vi "Record Single Channel.vi"() -> ()   [LabVIEW 2014]
uses:
  <vilib>/DAQmx/read.llb/DAQmx Read (Analog 1D DBL 1Chan NSamp).vi
  <vilib>/DAQmx/create/channels.llb/DAQmx Create Channel (AI-Voltage-Basic).vi
  <vilib>/DAQmx/configure/timing.llb/DAQmx Timing (Sample Clock).vi
panel:
  in  "Record time per file (s)":dbl
  out "x >= y?":bool
  in  "File name add to the end \n(height)":string="h300"
  out "Sampling rate after filtering (Hz)":dbl
  in  "Avg points":i32
  in  "Filter type":T1(ring)
  in  "avg time (s)":dbl
  out "x/y":dbl
  in  "stop":bool
  in  "Record time (s)":dbl=1000.0 format="%0.2f"
  in  "Tab Control":enum32{"Page 1", "Page 2", "PSD", "PSD 2"}(tab)
  out "Waveform Chart":dbl[](graph)
  out "Waveform Graph":dbl[](graph)
  out "XY Graph":T2(graph)
  out "Waveform Graph 2":dbl[][](graph)
  in  "Save?":bool
  in  "number of samples per channel":i32=200000
  in  "rate":dbl=200000.0 format="%0.2f"
  in  "Sampling range (V)":dbl=1.0 format="%0.2f"
  in  "physical channels":tag="Dev2/ai19"
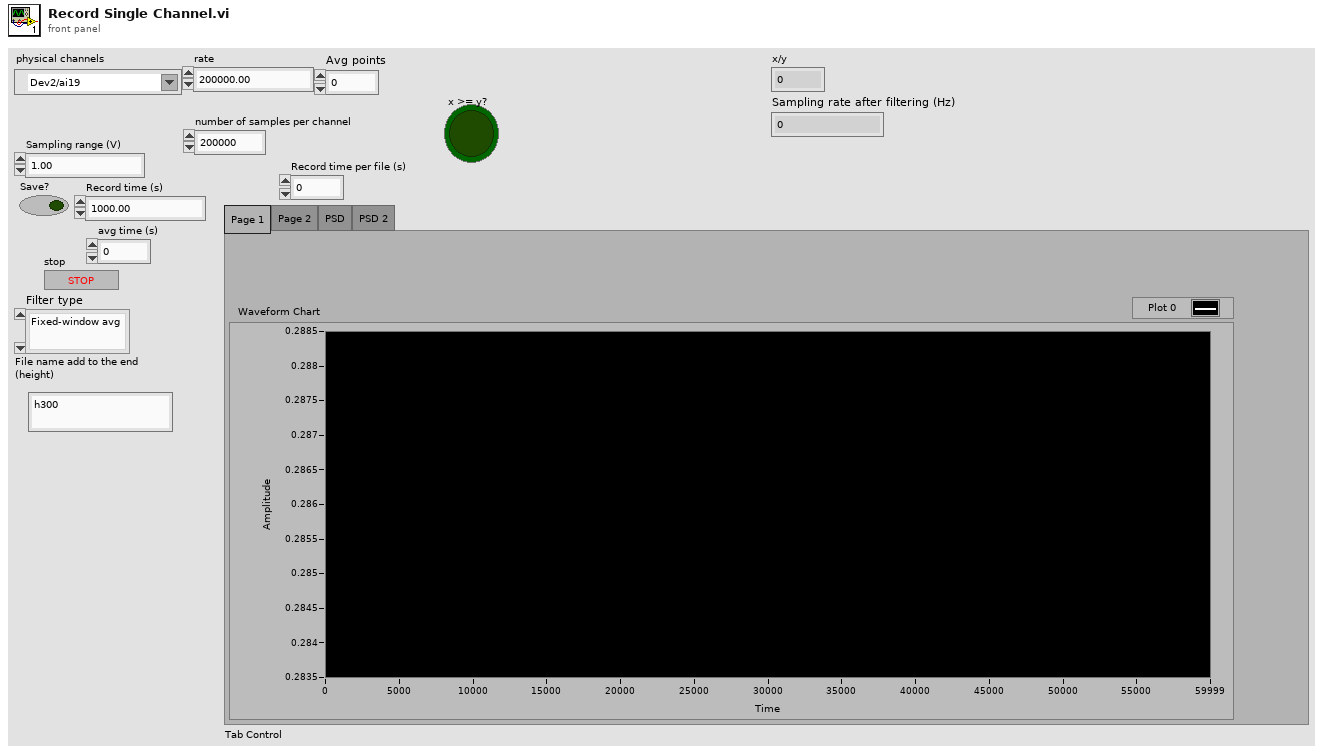
[diagram p1: front panel]
types:
  T1 = enum16{"Fixed-window avg", "Moving-window avg", "S-G filter", "Fixed-window Median", "Moving-window Median "}
  T2 = cluster{"Frequency (Hz)\n0,df, 2df,...(n/2-1)Fs":dbl[], "Avg. PSD":dbl[]}
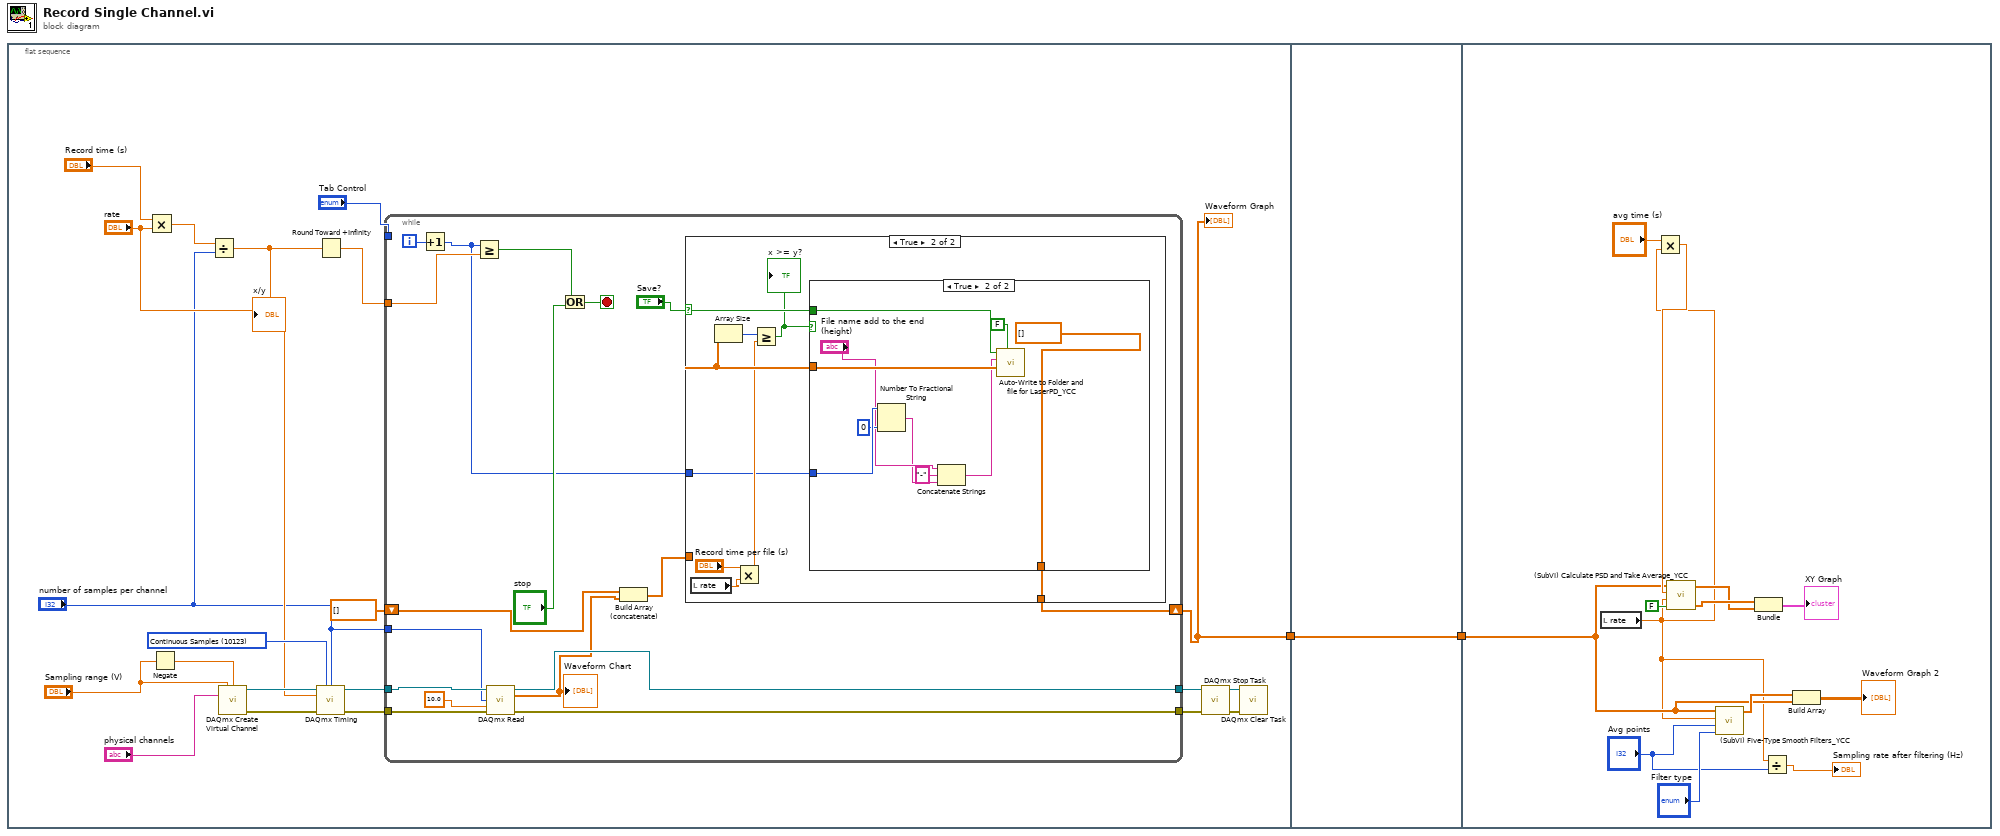
[diagram p0: block diagram]
diagram:
  n1 = flat-sequence {
    tunnel: [w3] -> w2
    tunnel: w2 -> [w62]
    tunnel: [w62] -> w1
    tunnel: w1 -> [w67]
    frame #0 {
      w18 = 10123 items=["Finite Samples"=10178, "Continuous Samples"=10123, "Hardware Timed Single Point"=12522] ("sample mode")
      n2 = Multiply(x="Record time (s)", y="rate") -> (x*y=w8:dbl)
      n3 = Negate(x="Sampling range (V)") -> (-x=w19:dbl)
      n4 = Divide(x=w8, y="number of samples per channel") -> (x/y=w7:dbl)
      "x/y" <- w7
      n5 = call-poly <vilib>:"DAQmx Create Virtual Channel.vi"("maximum value"="Sampling range (V)", "minimum value"=w19, "physical channels"="physical channels") -> ("task out"=w21:refnum<k21>, "error out"=w22:errorcluster)  [unwired: 11 in]
      n6 = Round Toward +Infinity(x=w7) -> (ceil(x): smallest int >= x=w6:dbl)
      n7 = call-poly <vilib>:"DAQmx Timing.vi"("task/channels in"=w21, "sample mode"=w18, "samples per channel"="number of samples per channel", "rate"="rate", "error in"=w22) -> ("task out"=w17:refnum<k21>, "error out"=w16:errorcluster)  [unwired: 9 in]
      n8 = while {
        tunnel: w17 -> [w40]
        tunnel: w16 -> [w39]
        tunnel: [w37] -> w15
        tunnel: [w36] -> w13
        tunnel: "Tab Control" -> [_]
        tunnel: w6 -> [w34]
        tunnel: "number of samples per channel" -> [w30]
        shift-right: [w25] -> w3
        shift-left: dbl[] [] -> [w28]
        i -> [w35]
        stop <- w31 stop-if-true
        n9 = Increment(x=w35) -> (x+1=w24:i32)
        n10 = Greater Or Equal?(x=w24, y=w34) -> (x >= y?=w33:bool)
        n11 = call-poly <vilib>:"DAQmx Read.vi"("task/channels in"=w40, "number of samples per channel"=w30, "timeout"=10.0, "error in"=w39) -> ("task out"=w37:refnum<k21>, "data"=w29:dbl[], "error out"=w36:errorcluster)  [unwired: 9 in]
        "Waveform Chart" <- w29
        n12 = Or(x=w33, y="stop") -> (x .or. y?=w31:bool)
        n13 = Build Array (concatenate)(w28, w29) -> (w26:dbl[])
        n14 = case shown="True" "Save?" {
          selector: "Save?" -> [_ w50]
          tunnel: w26 -> [w41 w48]
          tunnel: [w41 w49] -> w25
          tunnel: w24 -> [_ w42]
          frame False {
          }
          frame True {
            n15 = local read "rate"() -> (w45:dbl)
            n16 = Array Size(array=w48) -> (size(s)=w47:i32)
            n17 = Multiply(x="Record time per file (s)", y=w45) -> (x*y=w43:dbl)
            n18 = Greater Or Equal?(x=w47, y=w43) -> (x >= y?=w46:bool)
            "x >= y?" <- w46
            n19 = case shown="True" w46 {
              tunnel: w50 -> [_ w61]
              tunnel: w48 -> [w51 w60]
              tunnel: [w51 dbl[] []] -> w49
              tunnel: w42 -> [_ w57]
              frame False {
              }
              frame True {
                n20 = Number To Fractional String(number=w57, precision (6)=i16 0) -> (F-format string=w54:string)  [unwired: 2 in]
                n21 = Concatenate Strings("File name add to the end \n(height)", "-" ("string"), w54) -> (w52:string)
                n22 = call "Auto-Write to Folder and file for LaserPD_YCC.vi"("T=2D\nF=1D"=FALSE ("T=2D\nF=1D"), "1D data to be saved"=w60, "File name add to the end \n(height)"=w52, "Save?"=w61) -> ()  [unwired: 4 in, 2 out]
              }
            }
          }
        }
      }
      "Waveform Graph" <- w3
      n23 = call <vilib>:"DAQmx Stop Task.vi"("task/channels in"=w15, "error in"=w13) -> ("task out"=w14:refnum<k21>, "error out"=w12:errorcluster)  [unwired: 12 in]
      n24 = call <vilib>:"DAQmx Clear Task.vi"("task in"=w14, "error in"=w12) -> ()  [unwired: 13 in, 1 out]
    }
    frame #1 {
    }
    frame #2 {
      n25 = local read "rate"() -> (w63:dbl)
      n26 = Multiply(x="avg time (s)", y=w63) -> (x*y=w73:dbl)
      n27 = call "(SubVI) Calculate PSD and Take Average_YCC.vi"("Data"=w67, "#samples per avg"=w73, "Data rate (Hz)"=w63, "T=NI made PSD\nF=YCC made PSD"=FALSE ("T=NI made PSD\nF=YCC made PSD")) -> ("Avg. PSD"=w71:dbl[], "Frequency (Hz)\n0,df, 2df,...(n/2-1)Fs"=w72:dbl[])  [unwired: 3 in]
      n28 = call "(SubVI) Five-Type Smooth Filters_YCC.vi"("Filter type"="Filter type", "Avg points"="Avg points", "Sampling rate (Hz)"=w63, "QPD data"=w67) -> ("Filtered QPD data"=w68:dbl[])  [unwired: 1 in, 1 out]
      n29 = Bundle("Frequency (Hz)\n0,df, 2df,...(n/2-1)Fs"=w72, "Avg. PSD"=w71) -> (→"XY Graph":T2)  [unwired: 1 in]
      n30 = Divide(x=w63, y="Avg points") -> (x/y=→"Sampling rate after filtering (Hz)":dbl)
      n31 = Build Array(w68, w67) -> (→"Waveform Graph 2":dbl[][])
    }
  }
